vi "event density plot.vi"(8 "smoothing":i32, 9 "data in":dbl[](array[numeric])=array[52067 elements], 10 "data is sorted":bool, 11 "N":i32=200 min=0) -> (2 "data,sorted":dbl[](array[numeric]), 3 "Dynamic histogram out":T1(graph))   [LabVIEW 2019]
doc: "This VI generates an uneven spaced histogram that has N events and uses the width of the bins to calculate the event density. The event density is calculated using y[i] = N/(n[i+1]-n[i]) . The xa values are calculated using x[i] = (n[i]+n-[1+1])/2 . \nIn addition, smoothing can be applied. Smoothing can also be used to avoid zero progressin in subsequent bins that would otherwise result in devision by zero."
uses:
  <vilib>/Analysis/NI_AALPro.lvlib
panel:
  out "error out":errorcluster
  in  "error in":errorcluster caption="error out"
  # "Event Density Plot"
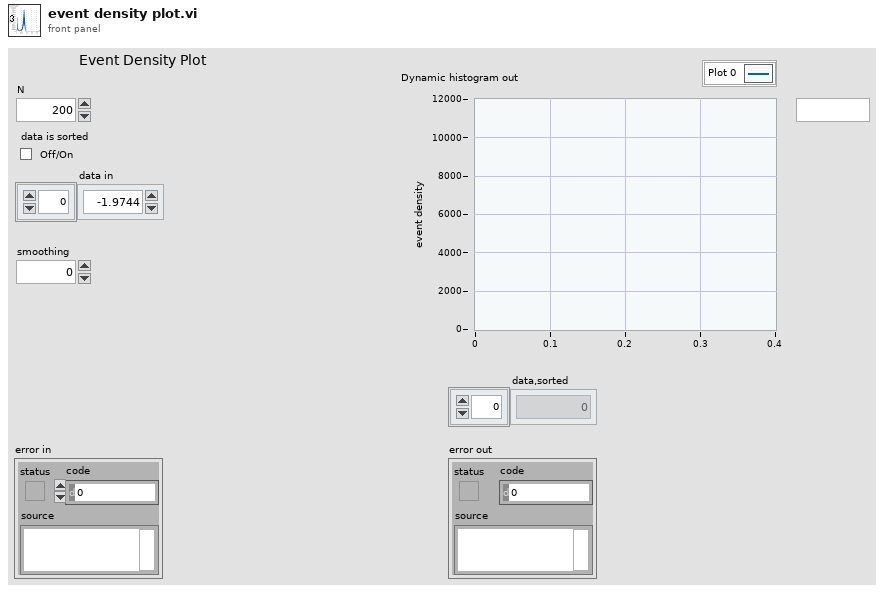
[diagram p1: front panel]
types:
  T1 = cluster{"Pulse amplitude":dbl[], "event density":dbl[]}
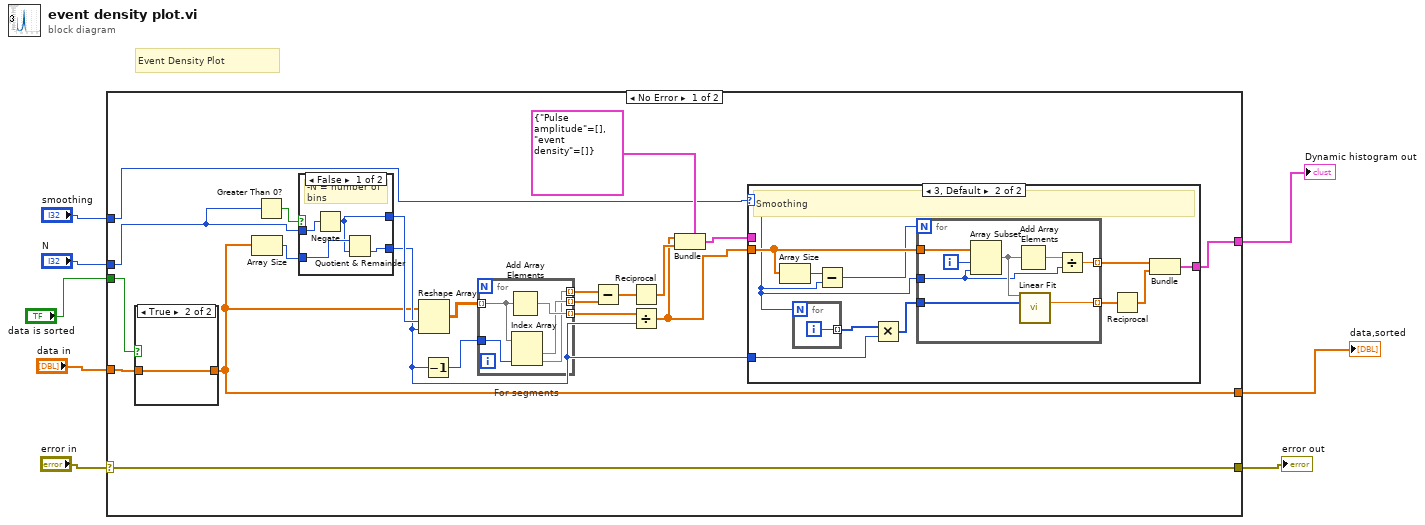
[diagram p0: block diagram]
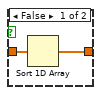
[diagram p3: hidden frame]
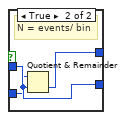
[diagram p4: hidden frame]
diagram:
  # "Event Density Plot"
  n1 = case shown="No Error" "error in" {
    selector: "error in" -> [w24 w66]
    tunnel: "N" -> [w21 _]
    tunnel: [w24 w66] -> w6
    tunnel: "data in" -> [w29 _]
    tunnel: [w15 _] -> w4
    tunnel: "smoothing" -> [w17 _]
    tunnel: [w10 _] -> w2
    tunnel: "data is sorted" -> [w9 _]
    frame No Error {
      n2 = case shown="True" w9 {
        tunnel: w29 -> [w52 w53]
        tunnel: [w51 w53] -> w10
        frame False {
          n3 = Sort 1D Array(array=w52) -> (sorted array=w51:dbl[])
        }
        frame True {
        }
      }
      n4 = Array Size(array=w10) -> (size(s)=w20:i32)
      n5 = Greater Than 0?(x=w21) -> (x > 0?=w22:bool)
      n6 = case shown="False" w22 {
        tunnel: w21 -> [w56 w60]
        tunnel: [w55 w60] -> w11
        tunnel: w20 -> [w57 w59]
        tunnel: [w54 w58] -> w19
        frame False {
          # "-N = number of bins"
          n7 = Negate(x=w56) -> (-x=w54:i32)
          n8 = Quotient & Remainder(x=w57, y=w54) -> (floor(x/y)=w55:i32)  [unwired: 1 out]
        }
        frame True {
          # "N = events/ bin"
          n9 = Quotient & Remainder(x=w59, y=w60) -> (floor(x/y)=w58:i32)  [unwired: 1 out]
        }
      }
      n10 = Reshape Array "Reshape Array"(w10, w19, w11) -> (w25:dbl[][])
      n11 = Decrement(x=w11) -> (x-1=w12:i32)
      n12 = for "For segments" {
        tunnel: w25 -> [w64] mode=indexing
        tunnel: [w65] -> w14 mode=indexing
        tunnel: [w63] -> w28 mode=indexing
        tunnel: w12 -> [w62]
        tunnel: [w61] -> w23 mode=indexing
        n13 = Add Array Elements(numeric array=w64) -> (sum=w65:dbl)
        n14 = Index Array(array=w64, index #2=w62) -> (element #1=w63:dbl, element #2=w61:dbl)  [unwired: 1 in]
      }
      n15 = Subtract(x=w23, y=w28) -> (x-y=w27:dbl[])
      n16 = Reciprocal(x=w27) -> (1/x=w26:dbl[])
      n17 = Divide(x=w14, y=w11) -> (x/y=w13:dbl[])
      n18 = Bundle(cluster=T1 {"Pulse amplitude"=[], "event density"=[]}, "Pulse amplitude"=w13, "event density"=w26) -> (w16:T1)
      n19 = case shown="3, Default" w17 {
        selector: w17 -> [_ w37]
        tunnel: w13 -> [_ w41]
        tunnel: w16 -> [w30 _]
        tunnel: [w30 w36] -> w15
        tunnel: w11 -> [_ w33]
        frame 0..2 {
          # "First implementation no smoothing"
        }
        frame 3, Default {
          # "Smoothing"
          n20 = Array Size(array=w41) -> (size(s)=w38:i32)
          n21 = for {
            N: w37 -> [_]
            tunnel: [w42] -> w32 mode=indexing
            i -> [w42]
          }
          n22 = Subtract(x=w38, y=w37) -> (x-y=w39:i32)
          n23 = Multiply(x=w32, y=w33) -> (x*y=w31:i32[])
          n24 = for {
            N: w39 -> [_]
            tunnel: w41 -> [w50]
            tunnel: [w49] -> w35 mode=indexing
            tunnel: w31 -> [w47]
            tunnel: [w44] -> w40 mode=indexing
            tunnel: w37 -> [w43]
            i -> [w48]
            n25 = Array Subset(array=w50, index=w48, length=w43) -> (w46:dbl[])
            n26 = Add Array Elements(numeric array=w46) -> (sum=w45:dbl)
            n27 = call <vilib>:"Linear Fit.vi"("Y"=w46, "X"=w47) -> ("slope"=w49:dbl)  [unwired: 9 in, 4 out]
            n28 = Divide(x=w45, y=w43) -> (x/y=w44:dbl)
          }
          n29 = Reciprocal(x=w35) -> (1/x=w34:dbl[])
          n30 = Bundle(w40, w34) -> (w36:cluster{dbl[], dbl[]})  [unwired: 1 in]
        }
      }
    }
    frame Error {
    }
  }
  "error out" <- w6
  "Dynamic histogram out" <- w4
  "data,sorted" <- w2
